vi "Load PS.vi"(11 "Path":path) -> (2 "Array":dbl[](array[numeric]), 3 "Array 2":dbl[](array[numeric]))   [LabVIEW 2018]
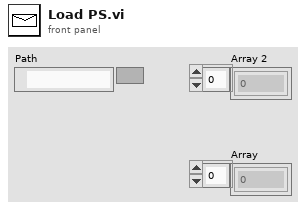
[diagram p1: front panel]
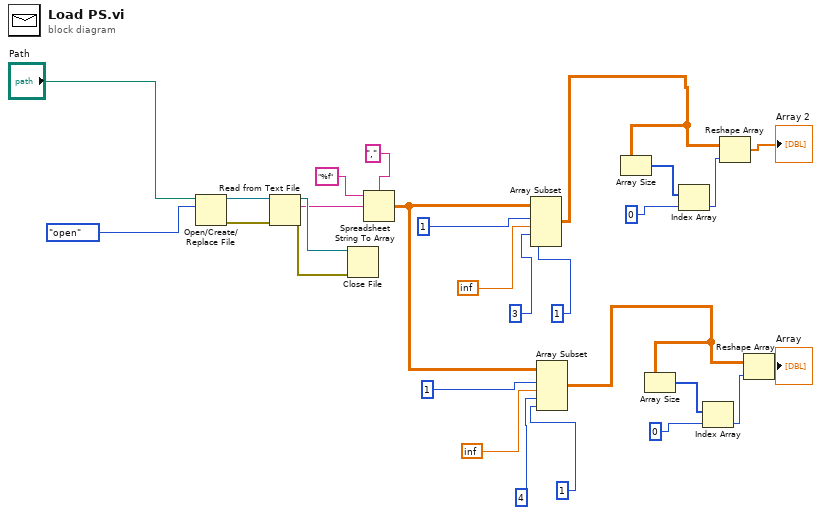
[diagram p0: block diagram]
diagram:
  n1 = Open/Create/Replace File(file path (use dialog)="Path", operation (0:open)=enum16{"open"}."open") -> (refnum out=w4:refnum<file>, error out=w3:errorcluster)  [unwired: 4 in, 1 out]
  n2 = Read from Text File(file (use dialog)=w4, error in=w3) -> (refnum out=w17:refnum<file>, text=w5:string, error out=w18:errorcluster)  [unwired: 2 in, 1 out]
  n3 = Close File(refnum=w17, error in=w18) -> ()  [unwired: 2 out]
  n4 = Spreadsheet String To Array(delimiter (Tab)=",", format string="%f", spreadsheet string=w5) -> (array=w14:dbl[][])  [unwired: 1 in]
  n5 = Array Subset(array=w14, index (row)=1, length (row)=inf, index (col)=3, length (col)=1) -> (w22:dbl[][])
  n6 = Array Subset(array=w14, index (row)=1, length (row)=inf, index (col)=4, length (col)=1) -> (w28:dbl[][])
  n7 = Array Size(array=w22) -> (size(s)=w20:i32[])
  n8 = Array Size(array=w28) -> (size(s)=w25:i32[])
  n9 = Index Array(array=w20, index=0) -> (element=w19:i32)
  n10 = Index Array(array=w25, index=0) -> (element=w24:i32)
  n11 = Reshape Array(w22, w19) -> (→"Array 2":dbl[])
  n12 = Reshape Array(w28, w24) -> (→"Array":dbl[])
